vi "setFlowRateSpec.vi"(2 "Flow Rate (sccm)":dbl, 3 "Flow range Index":T1 caption="Flow range" items=["0-10 sccm", "0-100 sccm", "0-1000 sccm"], 4 "D/A Card":T2={"Card Index"=0, "Channel Index"=3} {"Card Index" items=["Card 1", "Card 2", "Card 3", "Card 4", "Card 5", "Card 6"]; "Channel Index" items=["Channel 1", "Channel 2", "Channel 3", "Channel 4"]}) -> ()   [LabVIEW 2011]
uses:
  DA_Spec.ctl
  MFC_Spec.ctl
panel:
  out "x*y":dbl
  out "element":dbl
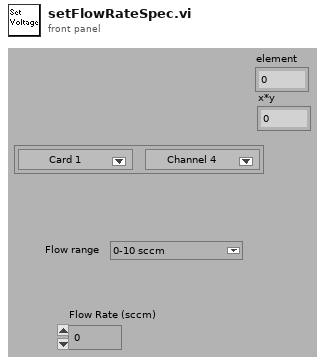
[diagram p1: front panel]
types:
  T1 = typedef "MFC_Spec.ctl" = u16
  T2 = typedef "DA_Spec.ctl" = cluster{"Card Index":u16, "Channel Index":u16}
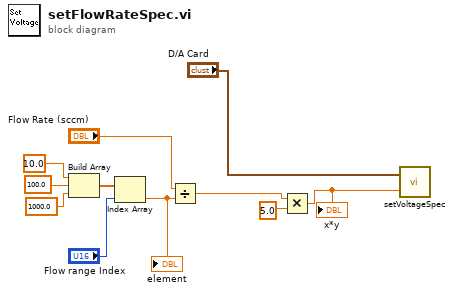
[diagram p0: block diagram]
diagram:
  n1 = Build Array(10.0 ("element"), 100.0 ("element"), 1000.0 ("element")) -> (w9:dbl[])
  n2 = Index Array(array=w9, index="Flow range Index") -> (element=w10:dbl)
  "element" <- w10
  n3 = Divide(x="Flow Rate (sccm)", y=w10) -> (x/y=w2:dbl)
  n4 = Multiply(x=w2, y=5.0) -> (x*y=w1:dbl)
  "x*y" <- w1
  n5 = call "setVoltageSpec.vi"("Voltage"=w1, "DA_Spec"="D/A Card") -> ()  [unwired: 1 in]
